vi "init.vi"(0 "ADC Channel0 Test in":refnum<class "ADC Channel0 Test.lvclass">, 1 "Signal Name":string, 2 "Test Scenario":T2, 3 "ILC Ch0 Analog Input Test":T1 {"PGA Gain Coefficients" max=7}, 4 "Samples To Average":i32, 5 "error in (no error)":errorcluster, 6 "Log":refnum<class "ITestLog.lvclass">, 7 "ILC":refnum<class "ILC.lvclass">, 9 "Delay Between Test Steps":u16) -> (14 "ADC Channel0 Test  out":refnum<class "ADC Channel0 Test.lvclass">, 19 "error out":errorcluster)   [LabVIEW 2015, in "ADC Channel0 Test.lvclass"]
uses:
  ADC Channel0 Test.lvclass
  Model/TestLog/ITestLog/ITestLog.lvclass
  Typedefs/TestScenarioTypes.ctl
  Typedefs/ILC Ch0 Analog Input Test.ctl
  <userlib>/Common/ILC/ILC/ILC.lvclass
  ADC Channel0 Test.lvclass/ADC Channel0 Test.ctl
  Typedefs/ILCBTTypedefs.lvlib
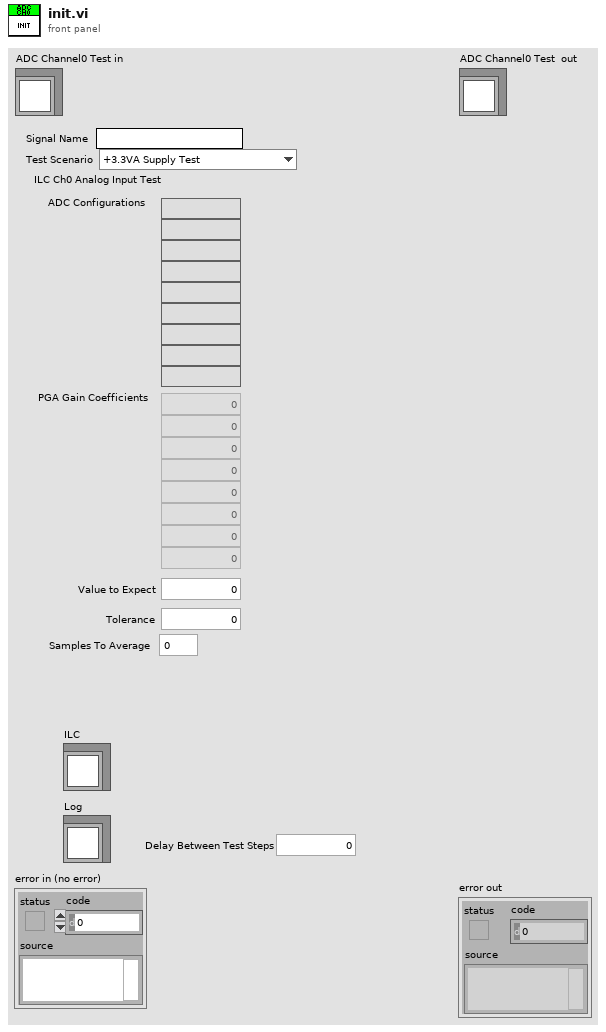
[diagram p1: front panel]
types:
  T1 = typedef "ILCBTTypedefs.lvlib/ILC Ch0 Analog Input Test.ctl" = cluster{"ADC Configurations":string[], "Value to Expect":i32, "Tolerance":i32, "PGA Gain Coefficients":u16[]}
  T2 = typedef "ILCBTTypedefs.lvlib/TestScenarioTypes.ctl" = enum16{"+3.3VA Supply Test", "+3.3VD Supply Test", "+5VA Supply Test", "+5VD Supply Test", "Unique ID Test", "TEDS Status Test", "LIMSW1_TTL Low Test", "LIMSW1_TTL High Test", "LIMSW2_TTL Low Test", "LIMSW2_TTL High Test", "Tachometer Low Test", "Tachometer High Test", "SSR_TTL Low Test", "SSR_TTL High Test", "SM_GPI Low Test", "SM_GPI High Test", "CW Motion Without Limit Test", "CW Motion With Limit Test", "CW Motion With Both Limits Test", "CW Motion on CCW Limit Test", "CCW Motion Without Limit Test", "CCW Motion With Limit Test", "CCW Motion With Both Limits Test", "CCW Motion on CW Limit Test", "RS232-TXD Low Test", "RS232-TXD High Test", "RS232-RTS Low Test", "RS232-RTS High Test", "RS232-RXD Low Test", "RS232-RXD High Test", "RS232-CTS Low Test", "RS232-CTS High Test", "Out_SS Low Test", "Out_SS High Test", "Out_SDI Low Test", "Out_SDI High Test", "Out_SCLK Low Test", "Out_SCLK High Test", "Reset Low Test", "Reset High Test", "1 Channel ADC Test", "3 Channel ADC Test", "5 Channel ADC Test", "Vref Test", "ROT Test", "DAC1 Test", "DAC2 Test", "DAC3 Test", "DAC4 Test", "BIAS Test", "EXC1 Test", "EXC2 Test", "EXC3 Test", "EXC4 Test"}
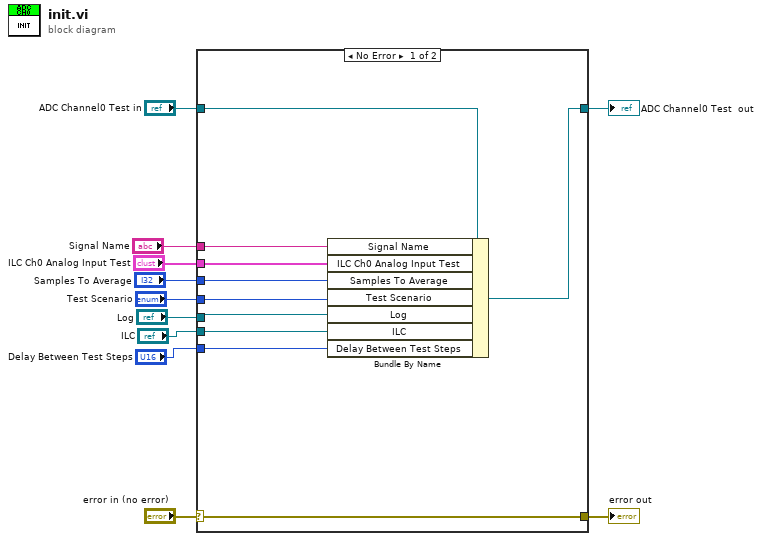
[diagram p0: block diagram]
diagram:
  n1 = case shown="No Error" "error in (no error)" {
    selector: "error in (no error)" -> [w21 w23]
    tunnel: [w21 w23] -> w10
    tunnel: [w20 w22] -> w8
    tunnel: "ADC Channel0 Test in" -> [w19 w22]
    tunnel: "Log" -> [w14 _]
    tunnel: "Signal Name" -> [w18 _]
    tunnel: "ILC Ch0 Analog Input Test" -> [w17 _]
    tunnel: "Samples To Average" -> [w16 _]
    tunnel: "Test Scenario" -> [w15 _]
    tunnel: "ILC" -> [w13 _]
    tunnel: "Delay Between Test Steps" -> [w12 _]
    frame No Error {
      n2 = Bundle By Name(cluster=w19, "Signal Name"=w18, "ILC Ch0 Analog Input Test"=w17, "Samples To Average"=w16, "Test Scenario"=w15, "Log"=w14, "ILC"=w13, "Delay Between Test Steps"=w12) -> (w20:refnum<class "ADC Channel0 Test.lvclass">)
    }
    frame Error {
    }
  }
  "error out" <- w10
  "ADC Channel0 Test  out" <- w8
